vi "3b - Read global.vi"() -> ()   [LabVIEW 2010]
uses:
  My Globals.vi
panel:
  out "Chart 2":dbl(graph)
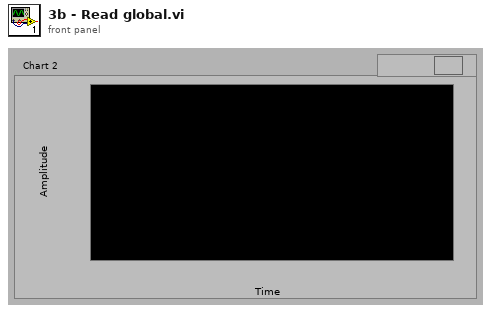
[diagram p1: front panel]
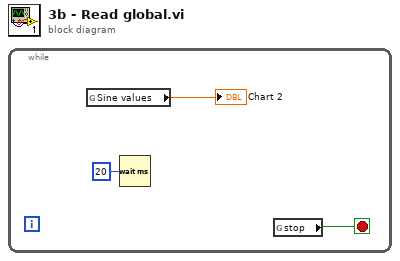
[diagram p0: block diagram]
diagram:
  n1 = while {
    stop <- w2 stop-if-true
    n2 = global read "My Globals.vi" "Sine values"() -> (→"Chart 2":dbl)
    n3 = Wait (ms)(milliseconds to wait=u32 20) -> ()  [unwired: 1 out]
    n4 = global read "My Globals.vi" "stop"() -> (w2:bool)
  }
